vi "Write Digital Output Port.vi"(8 "error in":errorcluster, 9 "Line grouping":T1(ring), 10 "data":u16, 11 "Write lines":string="Dev1/port0/line0") -> (0 "error out":errorcluster)   [LabVIEW 2013]
uses:
  <vilib>/DAQmx/create/channels.llb/DAQmx Create Channel (DO-Digital Output).vi
  <vilib>/DAQmx/write.llb/DAQmx Write (Digital U16 1Chan 1Samp).vi
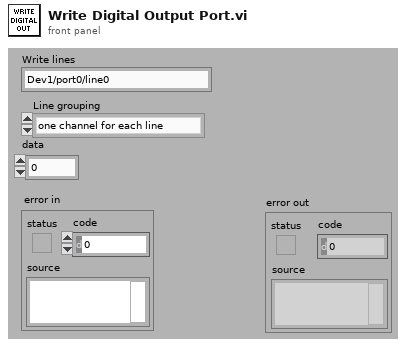
[diagram p1: front panel]
types:
  T1 = enum16{"one channel for each line", "one channel for all lines"}
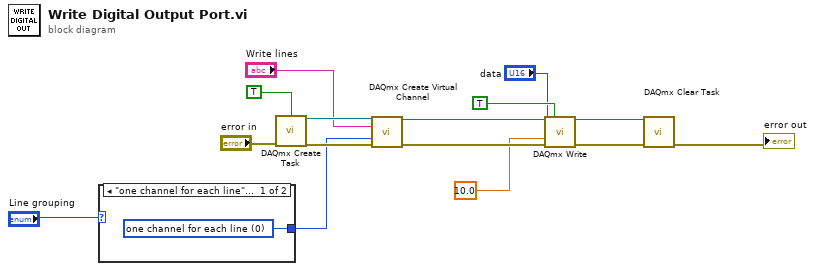
[diagram p0: block diagram]
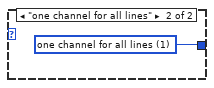
[diagram p2: hidden frame]
diagram:
  n1 = case shown="\"one channel for each line\", Default" "Line grouping" {
    tunnel: [w16 w17] -> w3
    frame "one channel for each line", Default {
      w16 = 0 items=["one channel for each line", "one channel for all lines"] ("line grouping")
    }
    frame "one channel for all lines" {
      w17 = 1 items=["one channel for each line", "one channel for all lines"] ("line grouping")
    }
  }
  n2 = call <vilib>:"DAQmx Create Task.vi"("auto cleanup"=TRUE, "error in"="error in") -> ("task out"=w12:refnum<k21>, "error out"=w13:errorcluster)  [unwired: 12 in]
  n3 = call-poly <vilib>:"DAQmx Create Virtual Channel.vi"("task in"=w12, "lines"="Write lines", "line grouping"=w3, "error in"=w13) -> ("task out"=w11:refnum<k21>, "error out"=w10:errorcluster)  [unwired: 10 in]
  n4 = call-poly <vilib>:"DAQmx Write.vi"("task/channels in"=w11, "auto start"=TRUE, "data"="data", "timeout"=10.0, "error in"=w10) -> ("task out"=w6:refnum<k21>, "error out"=w7:errorcluster)  [unwired: 8 in, 1 out]
  n5 = call <vilib>:"DAQmx Clear Task.vi"("task in"=w6, "error in"=w7) -> ("error out"=→"error out":errorcluster)  [unwired: 13 in]
